vi "Introspection Core.vi"(8 "error in (no error)":errorcluster, 11 "BNT_XtGraph in":refnum<class "BNT_XtGraph.lvclass">) -> (0 "error out":errorcluster, 2 "CSPP_Messages":refnum<class "Message.lvclass">[](array[class]), 3 "BNT_XtGraph out":refnum<class "BNT_XtGraph.lvclass">)   [LabVIEW 2018, in "BNT_XtGraph.lvlib" / "BNT_XtGraph.lvclass"]
doc: "This vi delivers a list with all messages this actor reacts to. \n\nNote that all inherited classes have to overwrite it."
uses:
  BNT_XtGraph.lvclass
  <vilib>/ActorFramework/Message/Message.lvclass
  BNT_XtGraph Messages/Add Data without TS Msg/Add Data without TS Msg.lvclass
  C:/Program Files (x86)/National Instruments/LabVIEW 2018/vi.lib/ActorFramework/Message/Message.lvclass
  CSPP_Core/Actors/CSPP_GUIActor/CSPP_GUIActor.lvclass
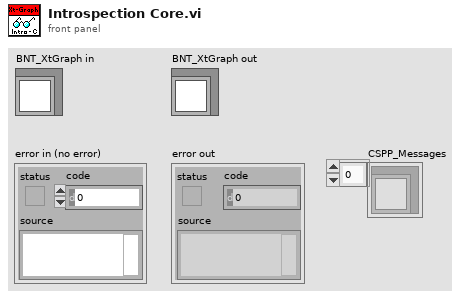
[diagram p1: front panel]
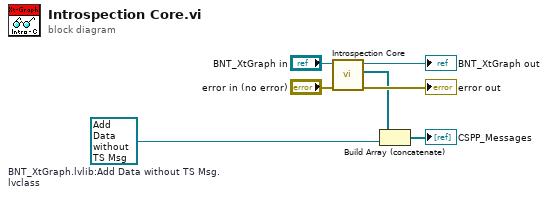
[diagram p0: block diagram]
diagram:
  w1 = refnum<class "Add Data without TS Msg.lvclass"> refnum  # BNT_XtGraph.lvlib:Add Data without TS Msg.lvclass
  n1 = call-parent "Introspection Core.vi"("error in (no error)"="error in (no error)", "CSPP_BaseActor in"="BNT_XtGraph in") -> ("error out"=→"error out":errorcluster, "CSPP_Messages"=w6:refnum<class "Message.lvclass">[], "CSPP_BaseActor out"=→"BNT_XtGraph out":refnum<class "BNT_XtGraph.lvclass">)  [unwired: 7 in]
  n2 = Build Array (concatenate)(w6, w1) -> (→"CSPP_Messages":refnum<class "Message.lvclass">[])
